vi "DoHandshake.vi"(0 "WebSocket Connection in":refnum<k5>, 5 "Supported Protocols (any)":string[](array[string]), 7 "Resource Names":string[](array[string]), 9 "timeout ms (5000)":i32=5000, 11 "error in (no error)":errorcluster, 12 "Additional Return headers (none)":T1[](array[typedef])) -> (4 "WebSocket Connection out":refnum<k5>, 6 "Headers Out":variant, 8 "Resource Name":string, 10 "Request URI":string, 14 "Host":string, 15 "error out":errorcluster)   [LabVIEW 2016, in "WebSockets.lvlib"]
doc: "Performs the WebSockets HTTP handshaking on the new TCP connection. The client sends HTTP headers and the server must reply with a correctly formed HTTP response. The VI handles an incoming WS-Protocol and will return it in the response headers if it matches the supported protocols input. Additional HTTP headers can also be returned.\nWebSockets 1.6.0.22\nSam Sharp - MediaMongrels Ltd\nCopyright (c) 2016, MediaMongrels Ltd"
uses:
  WebSockets.lvlib
  Headers.ctl
  HTTPResponseCodes.ctl
panel:
  out "HTTP Headers":string
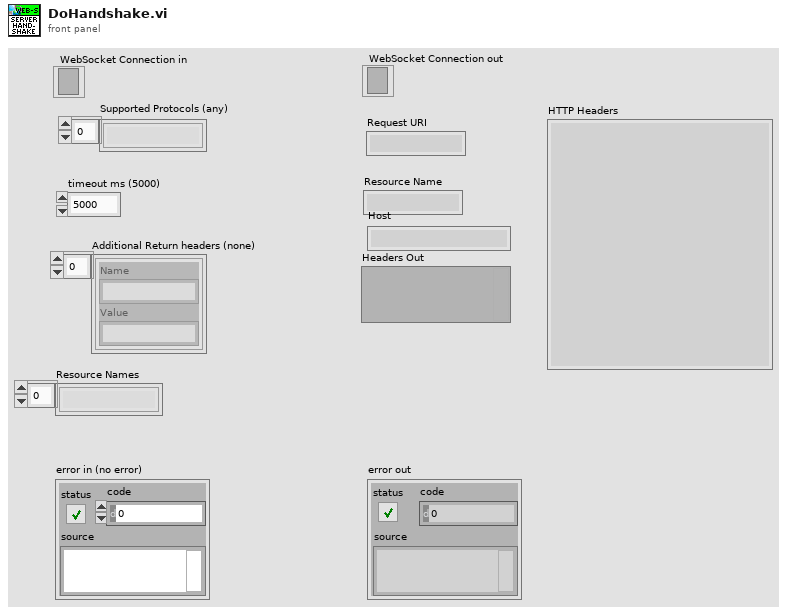
[diagram p1: front panel]
types:
  T1 = typedef "WebSockets.lvlib/Headers.ctl" = cluster{"Name":string, "Value":string}
  T2 = typedef "WebSockets.lvlib/HTTPResponseCodes.ctl" = u16
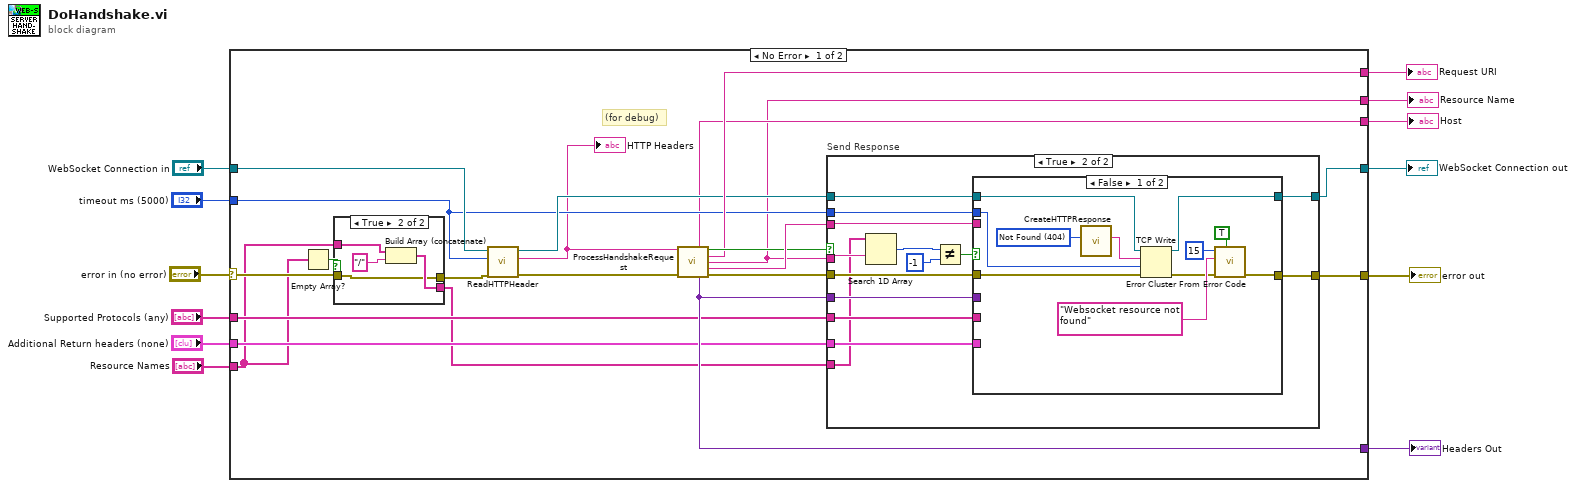
[diagram p0: block diagram]
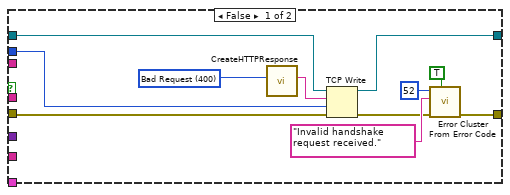
[diagram p3: hidden frame]
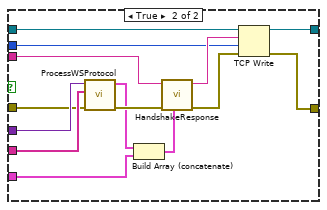
[diagram p4: hidden frame]
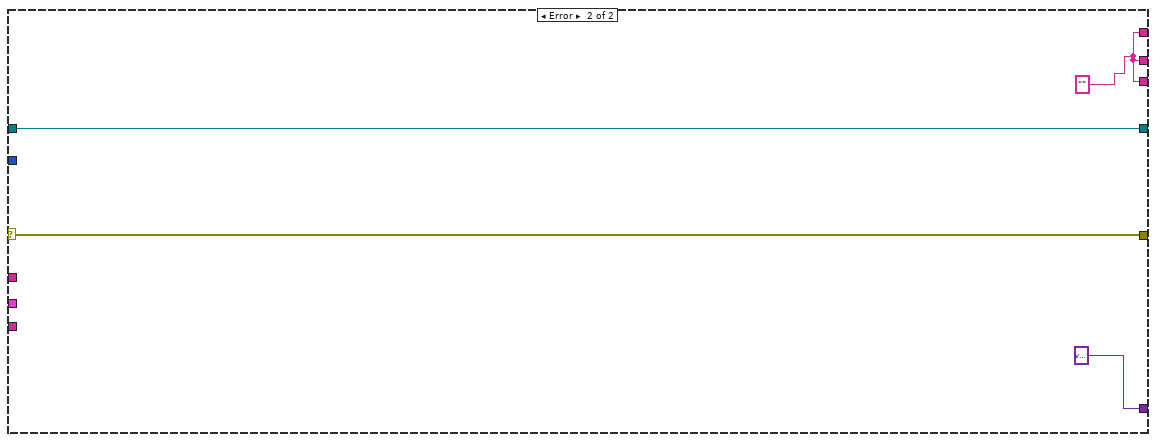
[diagram p5: hidden frame]
diagram:
  n1 = case shown="No Error" "error in (no error)" {
    selector: "error in (no error)" -> [w16 w93]
    tunnel: [w33 w92] -> w12
    tunnel: "WebSocket Connection in" -> [w27 w92]
    tunnel: [w29 w93] -> w9
    tunnel: "timeout ms (5000)" -> [w24 _]
    tunnel: [w22 variant ("Headers Out")] -> w7
    tunnel: [w28 w90] -> w6
    tunnel: "Supported Protocols (any)" -> [w21 _]
    tunnel: "Additional Return headers (none)" -> [w20 _]
    tunnel: [w18 w90] -> w3
    tunnel: [w19 w90] -> w2
    tunnel: "Resource Names" -> [w15 _]
    frame No Error {
      # "(for debug)"
      n2 = Empty Array?(array=w15) -> (empty?=w17:bool)
      n3 = case shown="True" w17 {
        tunnel: w16 -> [w34 w36]
        tunnel: [w35 w39] -> w14
        tunnel: w15 -> [w35 w37]
        tunnel: [w34 w36] -> w13
        frame False {
        }
        frame True {
          n4 = Build Array (concatenate)(w37, "/" ("name")) -> (w39:string[])
        }
      }
      n5 = call "ReadHTTPHeader.vi"("error in (no error)"=w13, "timeout ms (25000)"=w24, "WebSocket Connection in"=w27) -> ("error out"=w26:errorcluster, "HTTP Header"=w23:string, "WebSocket Connection out"=w25:refnum<k5>)  [unwired: 6 in]
      "HTTP Headers" <- w23
      n6 = call "ProcessHandshakeRequest.vi"("HTTP Headers"=w23, "error in (no error)"=w26) -> ("Host"=w19:string, "Is Websocket Request?"=w31:bool, "URI"=w28:string, "Resource Name"=w18:string, "Sec-WebSocket-Key"=w32:string, "Headers Out"=w22:variant, "error out"=w30:errorcluster)  [unwired: 7 in]
      n7 = case "Send Response" shown="True" w31 {
        tunnel: w32 -> [_ w64]
        tunnel: w25 -> [w41 w63]
        tunnel: [w40 w62] -> w33
        tunnel: w30 -> [w45 w55]
        tunnel: [w50 w61] -> w29
        tunnel: w24 -> [w42 w60]
        tunnel: w22 -> [_ w59]
        tunnel: w21 -> [_ w58]
        tunnel: w20 -> [_ w57]
        tunnel: w18 -> [_ w56]
        tunnel: w14 -> [_ w51]
        frame False {
          w46 = T2 400 items=["Switching Protocols"=101, "Bad Request"=400, "Forbidden"=403, "Not Found"=404, "Upgrade Required"=426] ("Http Response Codes")
          n8 = call "CreateHTTPResponse.vi"("Http Response Codes"=w46) -> ("Http Response"=w43:string)  [unwired: 10 in]
          n9 = TCP Write(connection ID=w41, data in=w43, error in (no error)=w45, 9:w42) -> (connection ID out=w40:refnum<k5>, error out=w44:errorcluster)  [unwired: 1 out]
          n10 = call <vilib>:"Error Cluster From Error Code.vi"("show call chain? (False)"=TRUE, "error in (no error)"=w44, "error message (\"\")"="Invalid handshake request received." ("error message (\"\")"), "error code (0)"=52) -> ("error out"=w50:errorcluster)  [unwired: 5 in]
        }
        frame True {
          n11 = Search 1D Array(1D array=w51, element=w56) -> (index of element=w53:i32)  [unwired: 1 in]
          n12 = Not Equal?(x=w53, y=-1) -> (x != y?=w54:bool)
          n13 = case shown="False" w54 {
            tunnel: w64 -> [_ w89]
            tunnel: w63 -> [w72 w87]
            tunnel: [w71 w86] -> w62
            tunnel: [w66 w84] -> w61
            tunnel: w60 -> [w70 w83]
            tunnel: w59 -> [_ w81]
            tunnel: w58 -> [_ w79]
            tunnel: w57 -> [_ w77]
            tunnel: w55 -> [w73 w76]
            frame False {
              w75 = T2 404 items=["Switching Protocols"=101, "Bad Request"=400, "Forbidden"=403, "Not Found"=404, "Upgrade Required"=426] ("Http Response Codes")
              n14 = call "CreateHTTPResponse.vi"("Http Response Codes"=w75) -> ("Http Response"=w74:string)  [unwired: 10 in]
              n15 = TCP Write(connection ID=w72, data in=w74, error in (no error)=w73, 9:w70) -> (connection ID out=w71:refnum<k5>, error out=w65:errorcluster)  [unwired: 1 out]
              n16 = call <vilib>:"Error Cluster From Error Code.vi"("show call chain? (False)"=TRUE, "error in (no error)"=w65, "error message (\"\")"="Websocket resource not found" ("error message (\"\")"), "error code (0)"=15) -> ("error out"=w66:errorcluster)  [unwired: 5 in]
            }
            frame True {
              n17 = call "ProcessWSProtocol.vi"("error in (no error)"=w76, "Supported Protocols (any)"=w79, "Headers In"=w81) -> ("error out"=w82:errorcluster, "Protocol Header"=w80:T1[])  [unwired: 7 in]
              n18 = Build Array (concatenate)(w80, w77) -> (w78:T1[])
              n19 = call "HandshakeResponse.vi"("additional headers (none)"=w78, "error in (no error)"=w82, "Sec-WebSocket-Key"=w89) -> ("error out"=w85:errorcluster, "Response Headers"=w88:string)  [unwired: 7 in]
              n20 = TCP Write(connection ID=w87, data in=w88, error in (no error)=w85, 9:w83) -> (connection ID out=w86:refnum<k5>, error out=w84:errorcluster)  [unwired: 1 out]
            }
          }
        }
      }
    }
    frame Error {
      w90 = "" ("Path")
    }
  }
  "WebSocket Connection out" <- w12
  "error out" <- w9
  "Headers Out" <- w7
  "Request URI" <- w6
  "Resource Name" <- w3
  "Host" <- w2
